vi "Check3DPointInsideBox.vi"(10 "3D Cuboid":T1, 11 "3D Point":T2) -> (3 "PointIsInsideCuboid":bool)   [LabVIEW 2020]
uses:
  3Dpoint.ctl
  3DCuboid.ctl
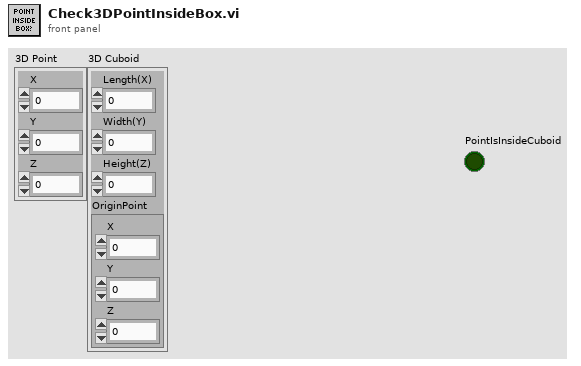
[diagram p1: front panel]
types:
  T1 = typedef "3DCuboid.ctl" = cluster{"Length(X)":dbl, "Width(Y)":dbl, "Height(Z)":dbl, "OriginPoint":T2}
  T2 = typedef "3Dpoint.ctl" = cluster{"X":dbl, "Y":dbl, "Z":dbl}
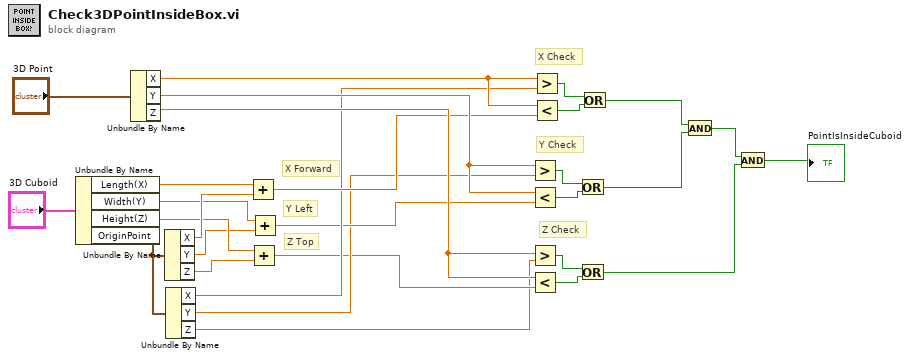
[diagram p0: block diagram]
diagram:
  # "X Check"
  # "Y Check"
  # "Z Check"
  # "Z Top"
  # "Y Left"
  # "X Forward"
  n1 = Unbundle By Name("3D Cuboid") -> ("Length(X)"=w27:dbl, "Width(Y)"=w23:dbl, "Height(Z)"=w24:dbl, "OriginPoint"=w6:T2)
  n2 = Unbundle By Name("3D Point") -> ("X"=w10:dbl, "Y"=w9:dbl, "Z"=w8:dbl)
  n3 = Unbundle By Name(w6) -> ("X"=w26:dbl, "Y"=w22:dbl, "Z"=w25:dbl)
  n4 = Unbundle By Name(w6) -> ("X"=w5:dbl, "Y"=w3:dbl, "Z"=w1:dbl)
  n5 = Add(x=w27, y=w26) -> (x+y=w7:dbl)
  n6 = Add(x=w24, y=w25) -> (x+y=w2:dbl)
  n7 = Add(x=w23, y=w22) -> (x+y=w4:dbl)
  n8 = Greater?(x=w9, y=w3) -> (0:w17:bool)
  n9 = Less?(x=w9, y=w4) -> (x < y?=w16:bool)
  n10 = Greater?(x=w8, y=w1) -> (0:w15:bool)
  n11 = Less?(x=w8, y=w2) -> (x < y?=w14:bool)
  n12 = Greater?(x=w10, y=w5) -> (0:w21:bool)
  n13 = Less?(x=w10, y=w7) -> (x < y?=w20:bool)
  n14 = Or(x=w17, y=w16) -> (x .or. y?=w12:bool)
  n15 = Or(x=w15, y=w14) -> (x .or. y?=w13:bool)
  n16 = Or(x=w21, y=w20) -> (x .or. y?=w11:bool)
  n17 = And(x=w11, y=w12) -> (x .and. y?=w18:bool)
  n18 = And(x=w18, y=w13) -> (x .and. y?=→"PointIsInsideCuboid":bool)
